vi "Multify(U8).vi"(1 "启用（T）":bool=TRUE, 2 "In":u8, 4 "n":u8=1) -> (6 "Out":u8=1)   [LabVIEW 2011]
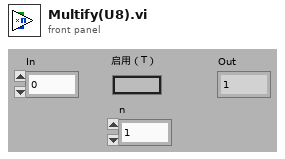
[diagram p1: front panel]
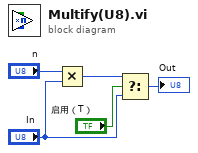
[diagram p0: block diagram]
diagram:
  n1 = Multiply(x="n", y="In") -> (x*y=w1:u8)
  n2 = Select(t=w1, s="启用（T）", f="In") -> (s? t:f=→"Out":u8)
